vi "adapt_image.vi"(5 "captured image?":bool, 6 "crop (TRUE)":bool=TRUE, 8 "captImage_Y_Resolution":i32, 9 "captImage_X_Resolution":i32, 11 "orig_imageIn":T1) -> (1 "adapted image px array":u8[][](array[numeric]), 3 "adapted image":T1)   [LabVIEW 2011]
doc: "Crops an image (original or captured) to cubic format (x-resolution = y-resolution) and applies a circular mask. Cropping and masking can be corrected using the crop-correction and mask-correction inputs.\n\nIf the input image is original (captured image set to FALSE) the image size will be adapted to match the size of the captured image and the image is flipped along the horizontal axis to account for the mirror image."
uses:
  <vilib>/vision/Image Controls.llb/IMAQ Image.ctl
  global_vars.vi
  <vilib>/vision/NI_Vision_Development_Module.lvlib
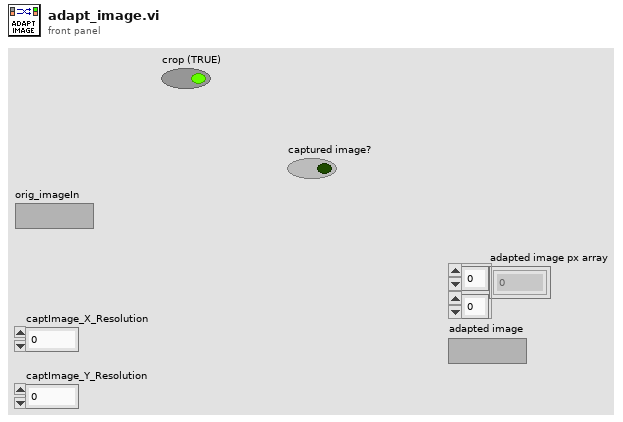
[diagram p1: front panel]
types:
  T1 = typedef "IMAQ Image.ctl" = refnum<image>
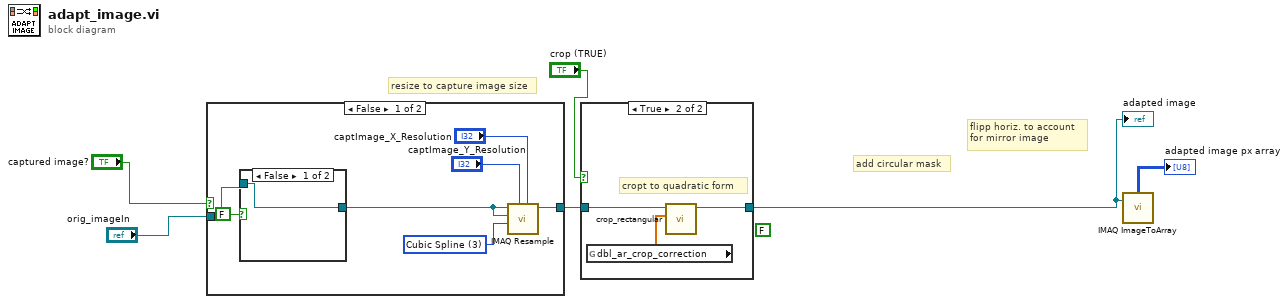
[diagram p0: block diagram]
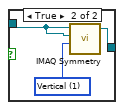
[diagram p3: hidden frame]
diagram:
  (unwired) FALSE
  # "flipp horiz. to account\nfor mirror image"
  # "resize to capture image size"
  # "add circular mask"
  n1 = case shown="False" "captured image?" {
    tunnel: [w11 w18] -> w6
    tunnel: "orig_imageIn" -> [w8 w18]
    frame False {
      w10 = u32 3 items=["Zero Order", "Bi-Linear", "Quadratic", "Cubic Spline"] ("Interpolation Type")
      n2 = case shown="False" FALSE {
        tunnel: [w14 w17] -> w9
        tunnel: w8 -> [w14 w15]
        frame False {
        }
        frame True {
          w16 = u32 1 items=["Horizontal", "Vertical", "Central", "1st Diagonal", "2nd Diagonal"] ("Type of Symmetry")
          n3 = call "IMAQ Symmetry"("Type of Symmetry"=w16, "Image Dst"=w15, "Image Src"=w15) -> ("Image Dst Out"=w17:T1)  [unwired: 2 in, 1 out]
        }
      }
      n4 = call "IMAQ Resample"("X Resolution"="captImage_X_Resolution", "Y Resolution"="captImage_Y_Resolution", "Interpolation Type"=w10, "Image Dst"=w9, "Image Src"=w9) -> ("Image Dst Out"=w11:T1)  [unwired: 5 in, 1 out]
    }
    frame True {
    }
  }
  n5 = case shown="True" "crop (TRUE)" {
    tunnel: w6 -> [w19 w22]
    tunnel: [w19 w21] -> w4
    frame False {
    }
    frame True {
      # "cropt to quadratic form"
      n6 = global read "global_vars.vi" "dbl_ar_crop_correction"() -> (w20:dbl[])
      n7 = call "crop_rectangular.vi"("dbl_ar_crop_correction"=w20, "image_in"=w22) -> ("cropped image out"=w21:T1)  [unwired: 8 in, 1 out]
    }
  }
  "adapted image" <- w4
  n8 = call "IMAQ ImageToArray"("Image"=w4) -> ("Image Pixels (U8)"=→"adapted image px array":u8[][])  [unwired: 3 in, 4 out]
